vi "FV_eval_current_turn.vi"(6 "valve_type":enum16{"Run", "Bypass"}(ring), 7 "backlash_corr":bool caption="Backlash Correction", 8 "error in":errorcluster, 11 "VISA":refnum<visa-resource-name>) -> (0 "error out":errorcluster, 1 "step_corr":i32, 2 "turn_now":dbl, 3 "VISA out":refnum<visa-resource-name>, 4 "status":bool, 5 "step_now":i32)   [LabVIEW 2019]
panel:
  out "step_rel_pre":i32
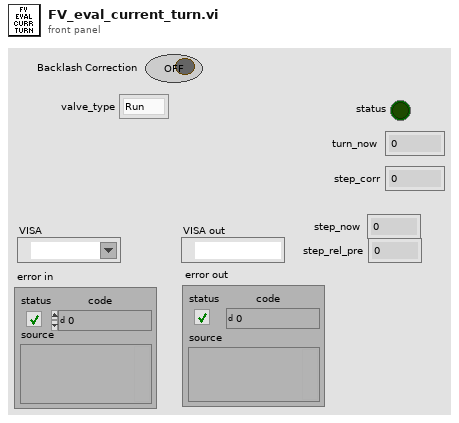
[diagram p1: front panel]
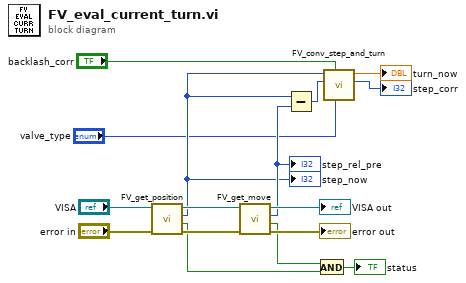
[diagram p0: block diagram]
diagram:
  n1 = call "FV_get_position.vi"("error in"="error in", "VISA"="VISA") -> ("error out"=w12:errorcluster, "status"=w1:bool, "Position"=w8:i32, "VISA out"=w14:refnum<visa-resource-name>)  [unwired: 6 in]
  "step_now" <- w8
  n2 = call "FV_get_move.vi"("error in"=w12, "VISA"=w14) -> ("error out"=→"error out":errorcluster, "status"=w2:bool, "step"=w9:i32, "VISA out"=→"VISA out":refnum<visa-resource-name>)  [unwired: 6 in]
  "step_rel_pre" <- w9
  n3 = Subtract(x=w8, y=w9) -> (x-y=w10:i32)
  n4 = And(x=w2, y=w1) -> (x .and. y?=→"status":bool)
  n5 = call "FV_conv_step_and_turn.vi"("valve_type"="valve_type", "backlash_corr"="backlash_corr", "step_in_pre"=w10, "step_in"=w8) -> ("step_corr_for_turn_out"=→"step_corr":i32, "turn_out"=→"turn_now":dbl)  [unwired: 4 in, 2 out]
